vi "Boiler.vi"() -> ()   [LabVIEW 2016]
uses:
  Controls/Boiler Controls.ctl
  Controls/Boiler Simulation Controls.ctl
  Controls/Boiler Status Indicators.ctl
  Controls/States.ctl
  <vilib>/Utility/file.llb/Write Delimited Spreadsheet (string).vi
panel:
  in  "Stop the Application":bool
  out "Boiler Status Indicators":T1 {"Time Count" format="%.2g"}
  in  "Boiler Simulation Controls":T2 {"Flame Sensor Value (%)" min=0.0 max=100.0 scale=0.0..100.0}
  in  "Boiler Controls":T3 {"Fuel Valve Position" min=0.0 max=100.0 scale=0.0..100.0 scale format="%.2f"}
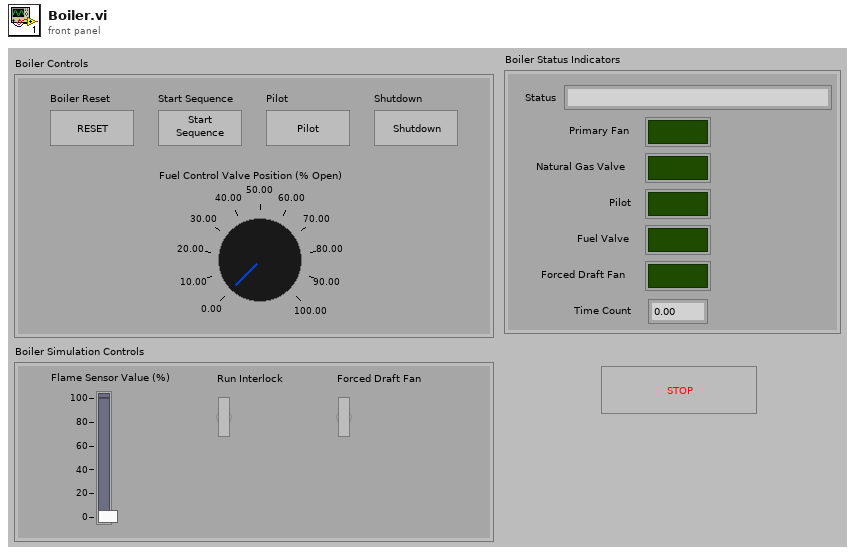
[diagram p1: front panel]
types:
  T1 = typedef "Boiler Status Indicators.ctl" = cluster{"Status":string, "Primary Fan":bool, "Natural Gas Valve":bool, "Pilot":bool, "Fuel Valve":bool, "Forced Draft Fan":bool, "Time Count":dbl}
  T2 = typedef "Boiler Simulation Controls.ctl" = cluster{"Flame Sensor Value (%)":dbl, "Run Interlock":bool, "Forced Draft Fan":bool}
  T3 = typedef "Boiler Controls.ctl" = cluster{"Boiler Reset":bool, "Start Sequence":bool, "Pilot":bool, "Shutdown":bool, "Fuel Valve Position":dbl}
  T4 = cluster{"Event string":string, "Event data string":string}
  T5 = typedef "States.ctl" = enum16{"Init", "Run", "Prove the Pilot", "Start and Run", "Shutdown"}
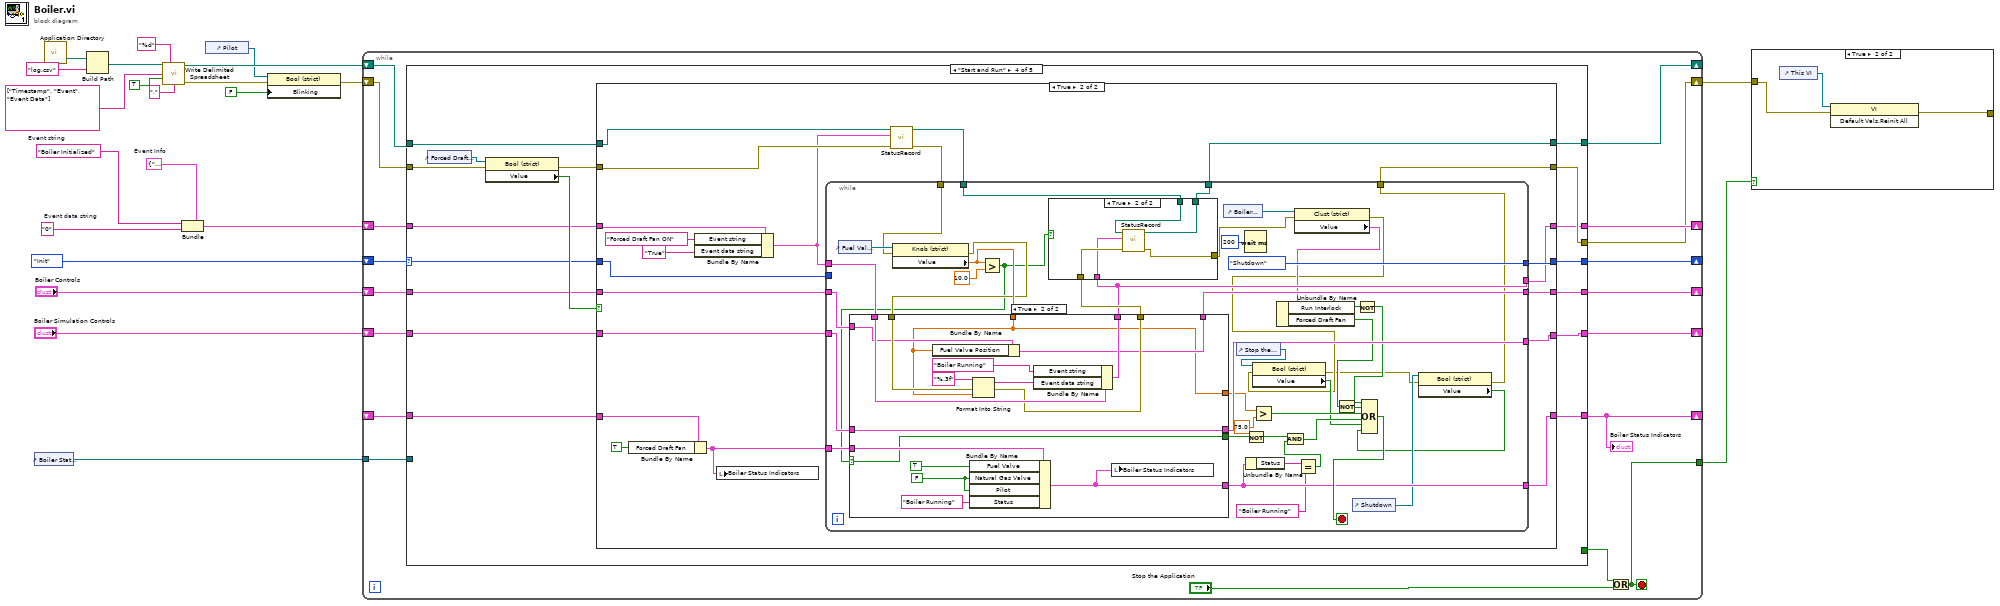
[diagram p0: block diagram]
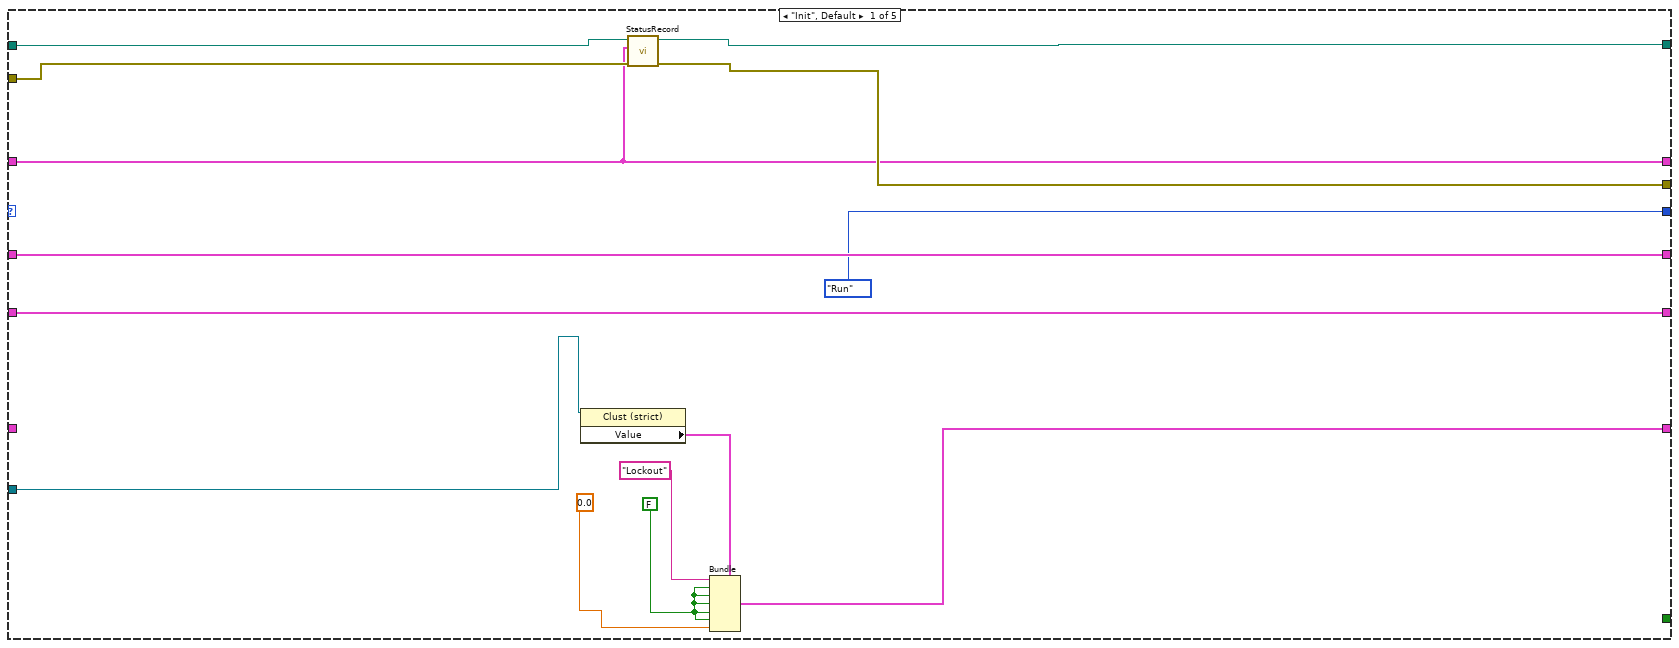
[diagram p3: hidden frame]
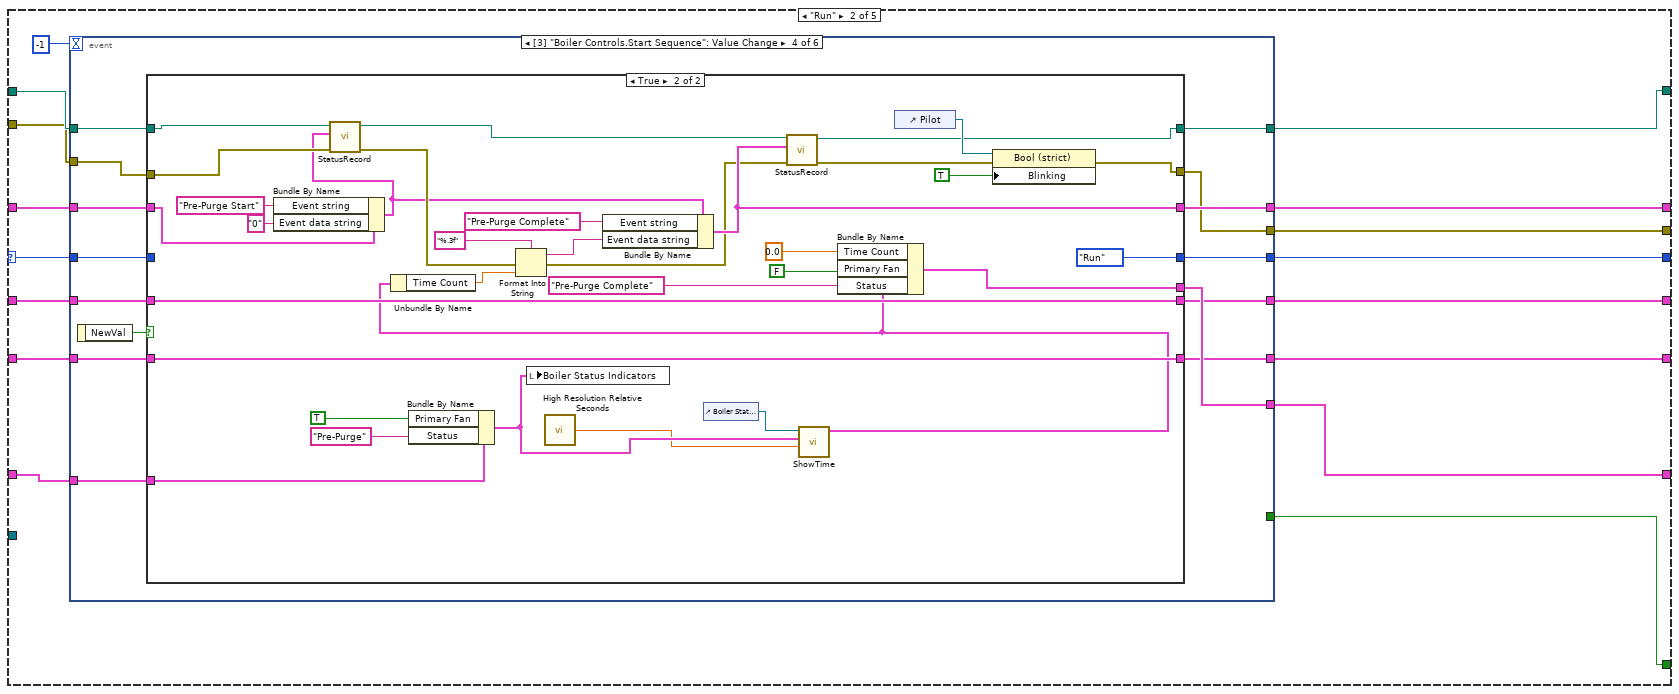
[diagram p4: hidden frame]
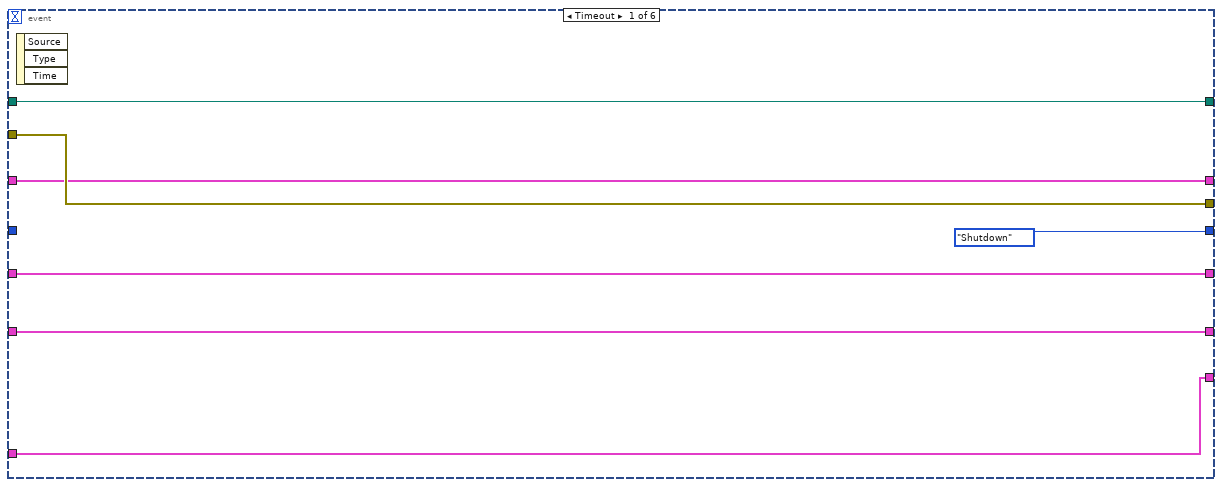
[diagram p5: hidden frame]
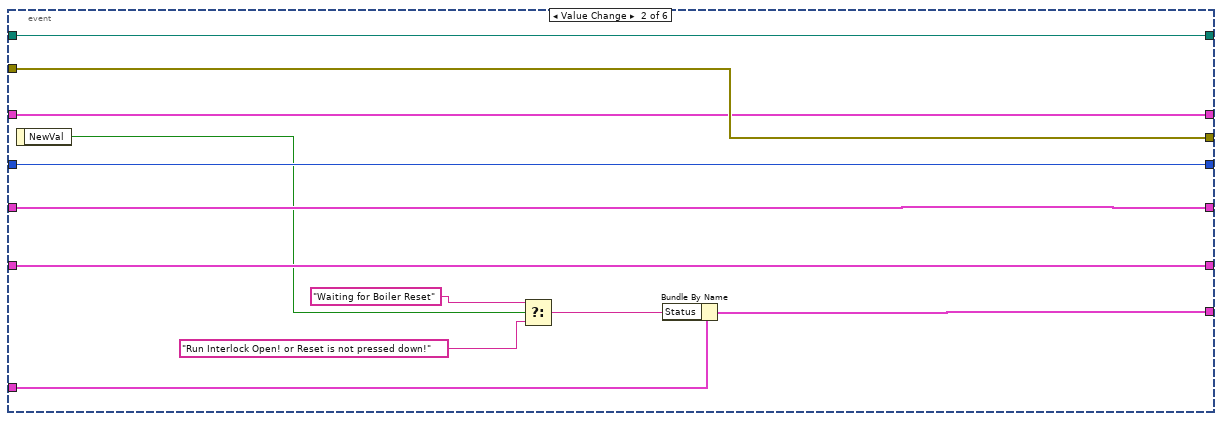
[diagram p6: hidden frame]
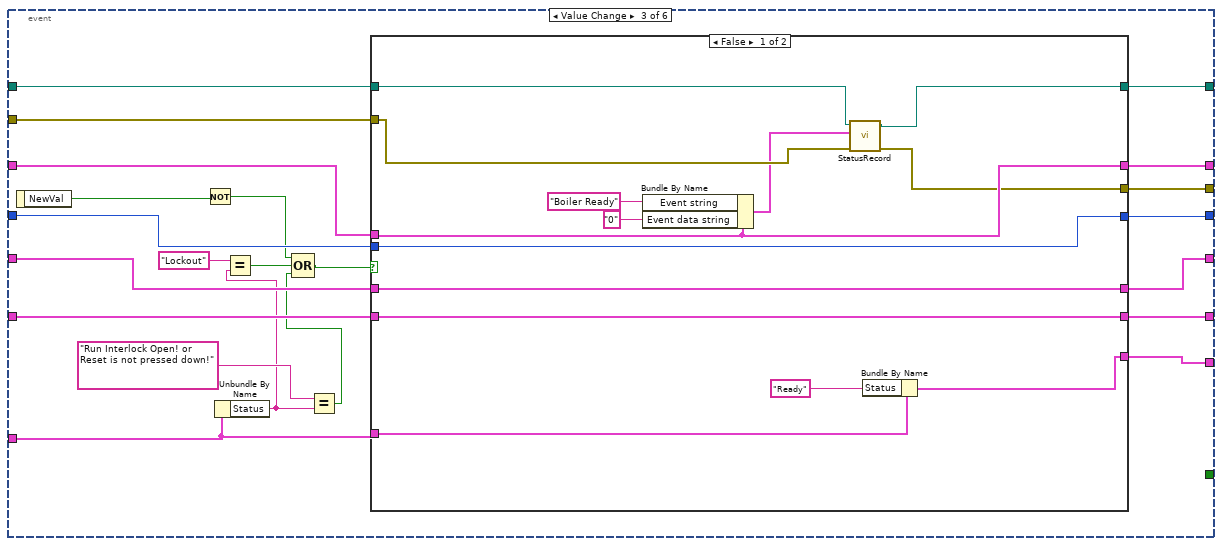
[diagram p7: hidden frame]
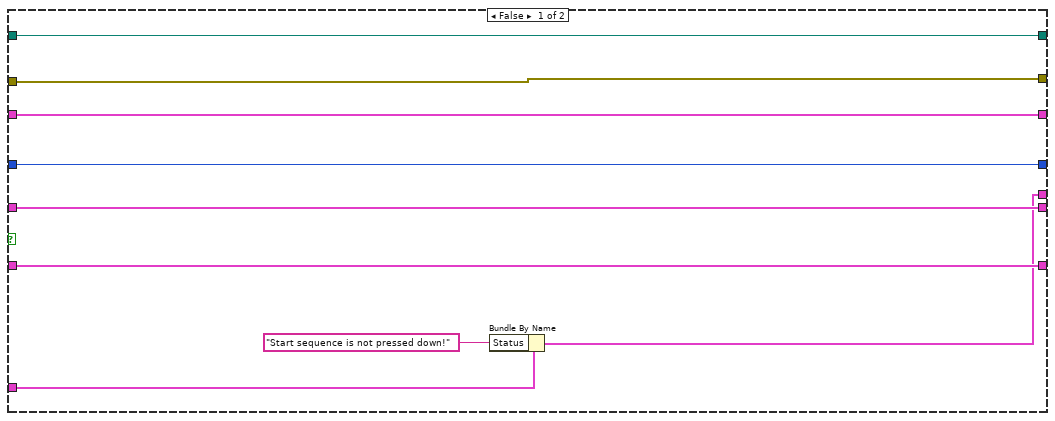
[diagram p9: hidden frame]
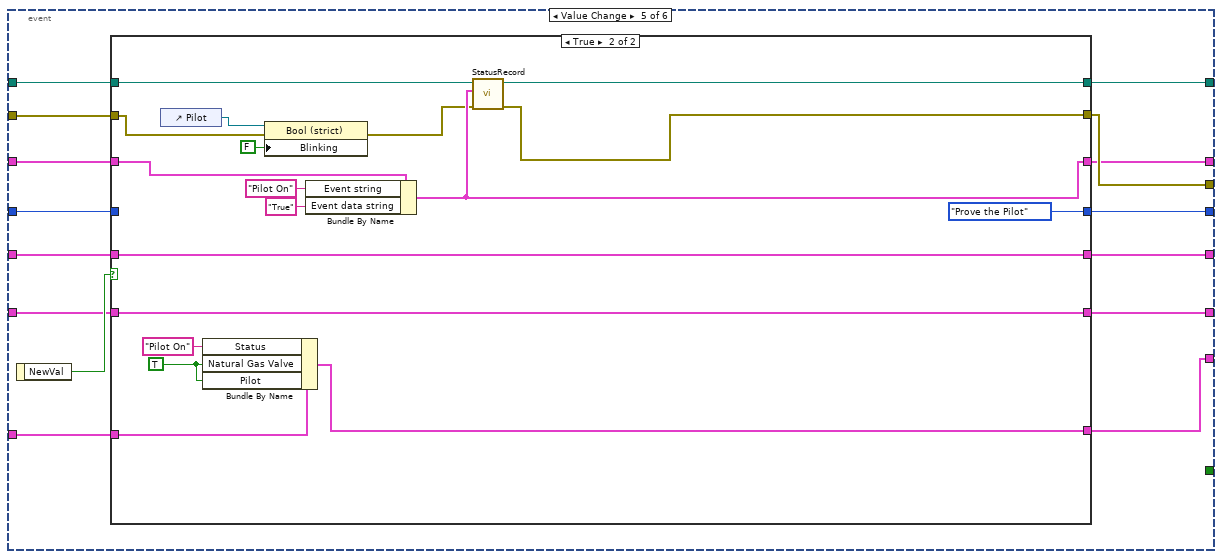
[diagram p10: hidden frame]
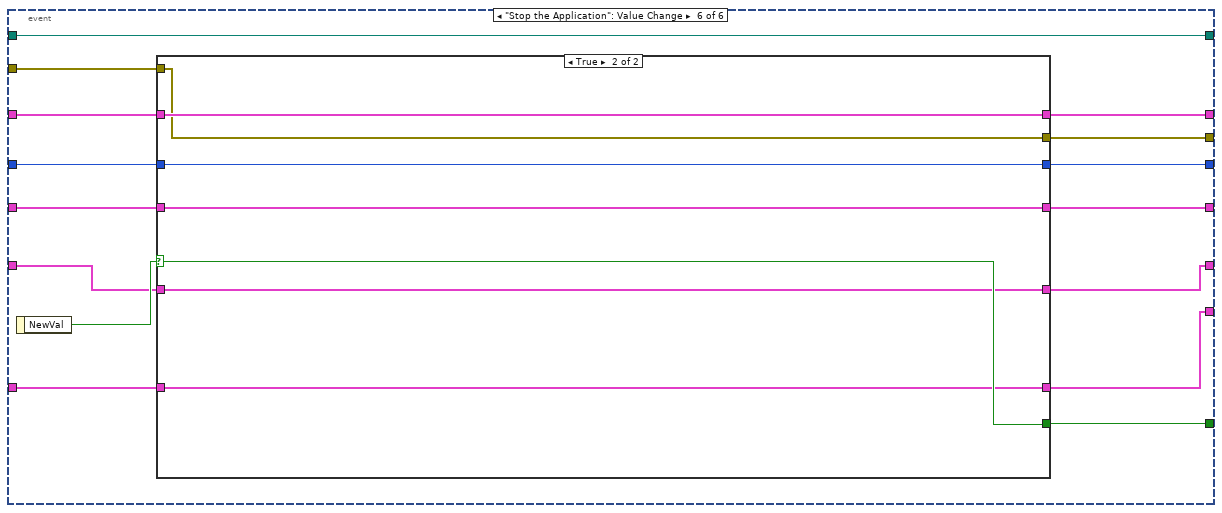
[diagram p12: hidden frame]
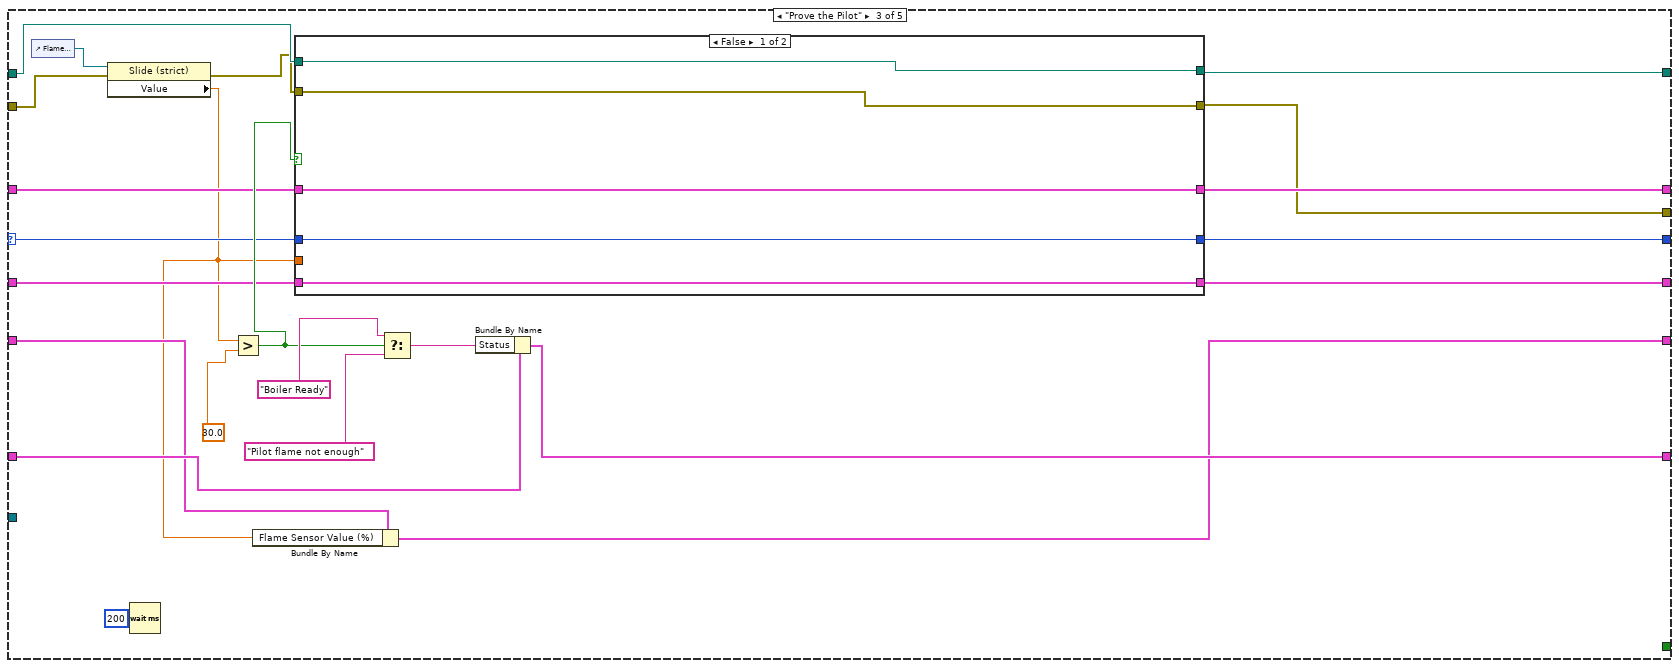
[diagram p14: hidden frame]
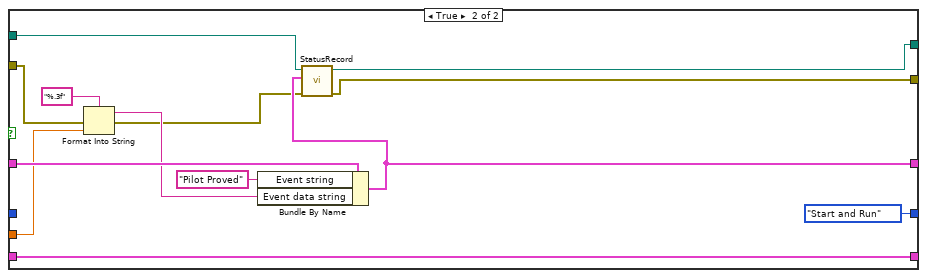
[diagram p15: hidden frame]
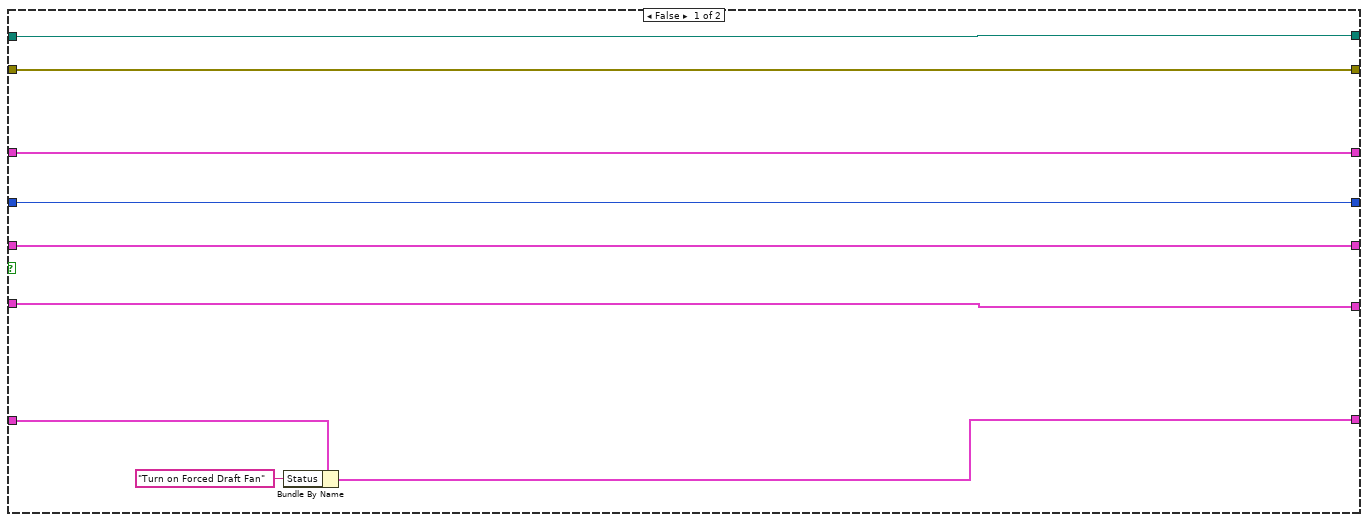
[diagram p16: hidden frame]
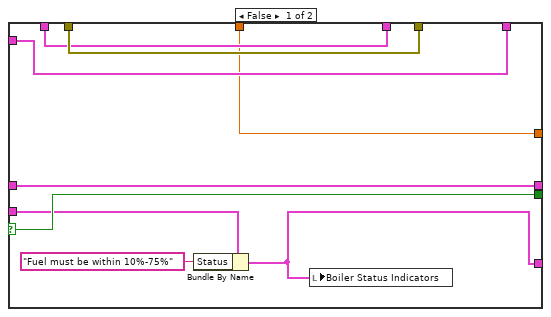
[diagram p18: hidden frame]
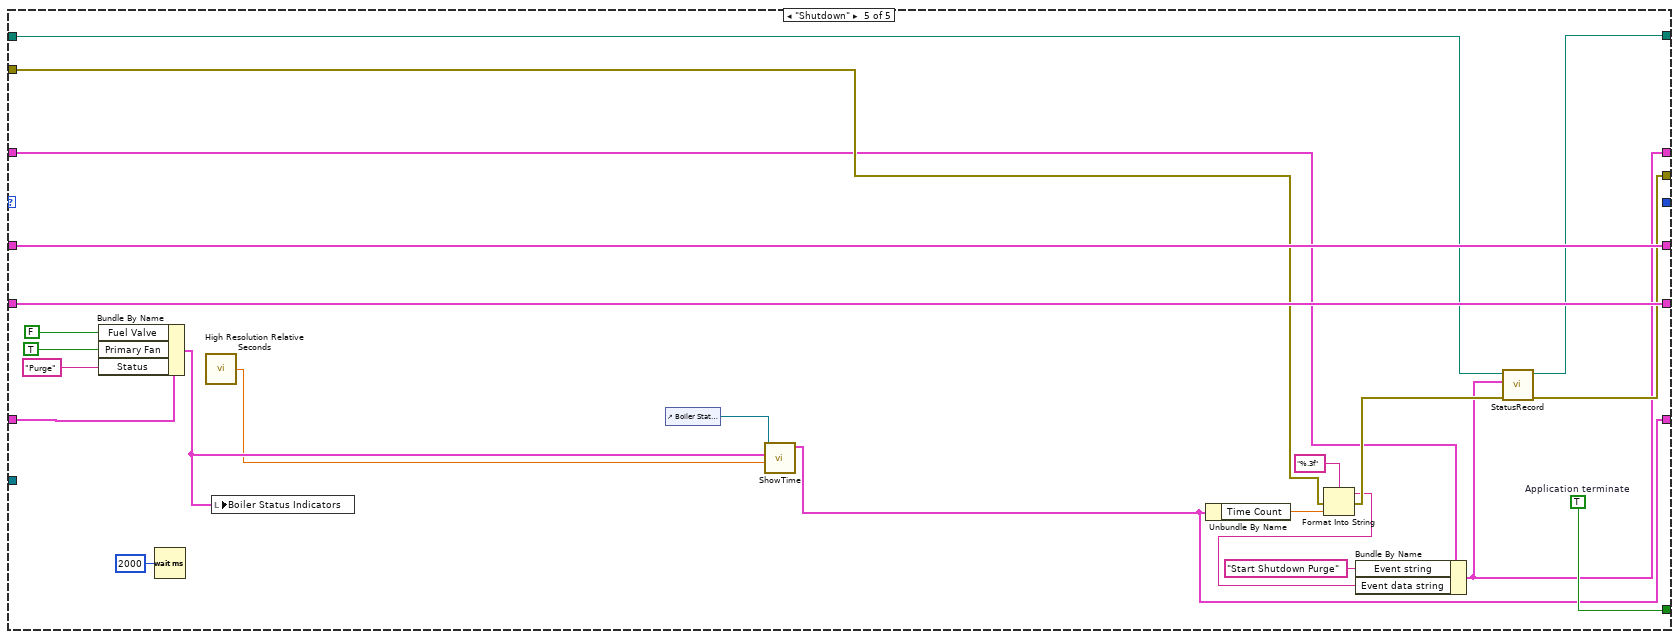
[diagram p19: hidden frame]
diagram:
  w7 = T4 {"Event string"="", "Event data string"=""}  # Event Info
  w17 = "Boiler Initialized"  # Event string
  w16 = "0"  # Event data string
  n1 = control-ref of="Boiler Status Indicators"() -> (w21:refnum<vi>)
  n2 = call <vilib>:"Application Directory.vi"() -> ("Application Directory"=w15:path)
  n3 = Build Path(base path=w15, name or relative path="log.csv") -> (appended path=w13:path)
  n4 = call-poly <vilib>:"Write Delimited Spreadsheet.vi"("file path (dialog if empty)"=w13, "format (%s)"="%d" ("format (%.3f)"), "1D data"=string[] ["Timestamp", "Event", "Event Data"], "append to file? (new file:F)"=TRUE, "delimiter (\\t)"="," ("delimiter (\\t)")) -> ("new file path (Not A Path if cancelled)"=w9:path, "error out"=w4:errorcluster)  [unwired: 9 in]
  n5 = Bundle(cluster=w7, "Event string"=w17, "Event data string"=w16) -> (w18:T4)
  n6 = control-ref of="Pilot"() -> (w5:refnum<vi>)
  n7 = property class="Bool (strict)"(reference=w5, error in=w4, "Blinking"=FALSE) -> (error out=w6:errorcluster)  [unwired: 1 out]
  n8 = while {
    tunnel: w21 -> [w39]
    shift-right: [w36] -> _
    shift-left: States."Init" -> [w40]
    shift-right: [w24] -> w2
    shift-left: w6 -> [w27]
    shift-right: [w34] -> _
    shift-left: w18 -> [w35]
    shift-right: [w31] -> _
    shift-left: "Boiler Controls" -> [w38]
    shift-right: [w32] -> _
    shift-left: "Boiler Simulation Controls" -> [w37]
    shift-right: [w25] -> _
    shift-left: _ -> [w30]
    shift-right: [w28] -> _
    shift-left: w9 -> [w29]
    tunnel: [w23] -> w1
    stop <- w23 stop-if-true
    n9 = case shown="\"Start and Run\"" w40 {
      selector: w40 -> [_ w64 w272 w307 _]
      tunnel: [w46 w59 w276 w300 w425] -> w25
      tunnel: w39 -> [w54 _ _ _ _]
      tunnel: w38 -> [w48 w65 w271 w305 w443]
      tunnel: w37 -> [w49 w66 w261 w303 w444]
      tunnel: [w49 w63 w259 w302 w444] -> w32
      tunnel: [w48 w62 w270 w304 w443] -> w31
      tunnel: [States."Run" w67 w269 w306 _] -> w36
      tunnel: [w44 w61 w266 w310 w427] -> w24
      tunnel: w27 -> [w45 w68 w264 w316 w432]
      tunnel: w35 -> [w41 w70 w273 w309 w430]
      tunnel: [w41 w60 w268 w308 w426] -> w34
      tunnel: [_ w57 _ _ w445] -> w33
      tunnel: w30 -> [_ w58 w278 w301 w439]
      tunnel: w29 -> [w43 w69 w274 w313 w429]
      tunnel: [w42 w55 w267 w312 w428] -> w28
      frame "Init", Default {
        w51 = FALSE ("Boiler Reset")
        n10 = property class="Clust (strict)"(reference=w54) -> ("Value"=w53:T1)  [unwired: 1 in, 2 out]
        n11 = call "StatusRecord.vi"("error in (no error)"=w45, "Event Info"=w41, "new file path (Not A Path if cancelled) in"=w43) -> ("error out"=w44:errorcluster, "new file path (Not A Path if cancelled) out"=w42:path)  [unwired: 7 in]
        n12 = Bundle(cluster=w53, "Status"="Lockout", "Primary Fan"=w51, "Natural Gas Valve"=w51, "Pilot"=w51, "Fuel Valve"=w51, "Forced Draft Fan"=w51, "Time Count"=0.0 ("Fuel Valve Position")) -> (w46:T1)
      }
      frame "Run" {
        n13 = event shown="[3] \"Boiler Controls.Start Sequence\": Value Change" {
          selector: _ -> [_ _ _ _ _ _]
          dyn-events: _ -> [_ _ _ _ _ _]
          timeout: -1 -> [_ _ _ _ _ _]
          tunnel: w70 -> [w74 w86 w102 w138 w199 w239]
          tunnel: w69 -> [w76 w88 w98 w135 w203 w242]
          tunnel: w68 -> [w75 w87 w100 w133 w201 w241]
          tunnel: [w76 w88 w97 w134 w202 w242] -> w55
          tunnel: [States."Shutdown" w85 w103 w139 w196 w236] -> w67
          tunnel: w66 -> [w72 w83 w108 w144 w193 w233]
          tunnel: w65 -> [w73 w84 w106 w142 w195 w235]
          tunnel: w58 -> [w71 w89 w110 w146 w191 w231]
          tunnel: [w71 w82 w109 w145 w190 w230] -> w59
          tunnel: w64 -> [_ w85 w104 w140 w197 w237]
          tunnel: [w72 w83 w107 w143 w192 w232] -> w63
          tunnel: [w73 w84 w105 w141 w194 w234] -> w62
          tunnel: [w75 w87 w99 w136 w200 w240] -> w61
          tunnel: [w74 w86 w101 w137 w198 w238] -> w60
          tunnel: [_ _ _ _ _ w243] -> w57
          event Timeout {
            n14 = event-data() -> ()  [unwired: 1 in, 3 out]
          }
          event Value Change {
            n15 = event-data() -> ("NewVal"=w81:bool)  [unwired: 1 in]
            n16 = Select(t="Waiting for Boiler Reset" ("Status"), s=w81, f="Run Interlock Open! or Reset is not pressed down!" ("Status")) -> (s? t:f=w78:string)
            n17 = Bundle By Name(cluster=w89, "Status"=w78) -> (w82:T1)
          }
          event Value Change {
            n18 = event-data() -> ("NewVal"=w96:bool)  [unwired: 1 in]
            n19 = Not(x=w96) -> (.not. x?=w95:bool)
            n20 = Unbundle By Name(w110) -> ("Status"=w93:string)
            n21 = Equal?(x="Lockout", y=w93) -> (x = y?=w91:bool)
            n22 = Equal?(x="Run Interlock Open! or Reset is not pressed down!" ("Status"), y=w93) -> (x = y?=w94:bool)
            n23 = Compound Arithmetic op=OR(w95, w91, w94) -> (w90:bool)
            n24 = case shown="False" w90 {
              tunnel: w110 -> [w122 w126]
              tunnel: [w118 w126] -> w109
              tunnel: w108 -> [w121 w127]
              tunnel: [w121 w127] -> w107
              tunnel: w106 -> [w120 w128]
              tunnel: [w120 w128] -> w105
              tunnel: w104 -> [w117 w129]
              tunnel: [w117 w129] -> w103
              tunnel: w102 -> [w119 w130]
              tunnel: [w119 w130] -> w101
              tunnel: w100 -> [w114 w131]
              tunnel: [w115 w131] -> w99
              tunnel: w98 -> [w113 w132]
              tunnel: [w116 w132] -> w97
              frame False {
                n25 = Bundle By Name(cluster=w119, "Event string"="Boiler Ready", "Event data string"="0") -> (w112:T4)
                n26 = call "StatusRecord.vi"("error in (no error)"=w114, "Event Info"=w112, "new file path (Not A Path if cancelled) in"=w113) -> ("error out"=w115:errorcluster, "new file path (Not A Path if cancelled) out"=w116:path)  [unwired: 7 in]
                n27 = Bundle By Name(cluster=w122, "Status"="Ready") -> (w118:T1)
              }
              frame True {
              }
            }
          }
          event Value Change {
            n28 = event-data() -> ("NewVal"=w147:bool)  [unwired: 1 in]
            n29 = case shown="True" w147 {
              tunnel: w146 -> [w155 w187]
              tunnel: [w148 w175] -> w145
              tunnel: w144 -> [w154 w186]
              tunnel: [w154 w186] -> w143
              tunnel: w142 -> [w153 w185]
              tunnel: [w153 w185] -> w141
              tunnel: w140 -> [w152 _]
              tunnel: [w152 States."Run"] -> w139
              tunnel: [w151 w163] -> w137
              tunnel: w138 -> [w151 w178]
              tunnel: [w150 w170] -> w136
              tunnel: w133 -> [w150 w158]
              tunnel: [w149 w165] -> w134
              tunnel: w135 -> [w149 w161]
              frame False {
                n30 = Bundle By Name(cluster=w155, "Status"="Start sequence is not pressed down!") -> (w148:T1)
              }
              frame True {
                n31 = Bundle By Name(cluster=w178, "Event string"="Pre-Purge Start", "Event data string"="0") -> (w157:T4)
                n32 = call "StatusRecord.vi"("error in (no error)"=w158, "Event Info"=w157, "new file path (Not A Path if cancelled) in"=w161) -> ("error out"=w159:errorcluster, "new file path (Not A Path if cancelled) out"=w160:path)  [unwired: 7 in]
                n33 = Bundle By Name(cluster=w187, "Primary Fan"=TRUE, "Status"="Pre-Purge") -> (w168:T1)
                n34 = local write "Boiler Status Indicators"(w168) -> ()
                n35 = call <vilib>:"High Resolution Relative Seconds.vi"() -> ("relative seconds"=w167:dbl)
                n36 = control-ref of="Boiler Status Indicators"() -> (w169:refnum<vi>)
                n37 = call "ShowTime.vi"("relative seconds"=w167, "Value in"=w168, "Cluster in"=w169) -> ("Value out"=w166:T1)  [unwired: 8 in]
                n38 = Unbundle By Name(w166) -> ("Time Count"=w182:dbl)
                n39 = Format Into String(format string="%.3f", error in=w159, w182) -> (resulting string=w180:string, error out=w162:errorcluster)  [unwired: 1 in]
                n40 = Bundle By Name(cluster=w157, "Event string"="Pre-Purge Complete", "Event data string"=w180) -> (w163:T4)
                n41 = call "StatusRecord.vi"("error in (no error)"=w162, "Event Info"=w163, "new file path (Not A Path if cancelled) in"=w160) -> ("error out"=w164:errorcluster, "new file path (Not A Path if cancelled) out"=w165:path)  [unwired: 7 in]
                n42 = Bundle By Name(cluster=w166, "Time Count"=0.0, "Primary Fan"=FALSE, "Status"="Pre-Purge Complete") -> (w175:T1)
                n43 = control-ref of="Pilot"() -> (w172:refnum<vi>)
                n44 = property class="Bool (strict)"(reference=w172, error in=w164, "Blinking"=TRUE) -> (error out=w170:errorcluster)  [unwired: 1 out]
              }
            }
          }
          event Value Change {
            n45 = event-data() -> ("NewVal"=w204:bool)  [unwired: 1 in]
            n46 = case shown="True" w204 {
              tunnel: [w211 w212] -> w202
              tunnel: w203 -> [w211 w216]
              tunnel: [w210 w213] -> w200
              tunnel: w201 -> [w210 w227]
              tunnel: [w209 w215] -> w198
              tunnel: w199 -> [w209 w220]
              tunnel: [w205 States."Prove the Pilot"] -> w196
              tunnel: w197 -> [w205 _]
              tunnel: [w208 w219] -> w194
              tunnel: w195 -> [w208 w219]
              tunnel: [w207 w218] -> w192
              tunnel: w193 -> [w207 w218]
              tunnel: [w206 w224] -> w190
              tunnel: w191 -> [w206 w226]
              frame False {
              }
              frame True {
                w225 = TRUE ("Natural Gas Valve")
                n47 = control-ref of="Pilot"() -> (w229:refnum<vi>)
                n48 = Bundle By Name(cluster=w226, "Status"="Pilot On", "Natural Gas Valve"=w225, "Pilot"=w225) -> (w224:T1)
                n49 = property class="Bool (strict)"(reference=w229, error in=w227, "Blinking"=FALSE) -> (error out=w214:errorcluster)  [unwired: 1 out]
                n50 = Bundle By Name(cluster=w220, "Event string"="Pilot On", "Event data string"="True") -> (w215:T4)
                n51 = call "StatusRecord.vi"("error in (no error)"=w214, "Event Info"=w215, "new file path (Not A Path if cancelled) in"=w216) -> ("error out"=w213:errorcluster, "new file path (Not A Path if cancelled) out"=w212:path)  [unwired: 7 in]
              }
            }
          }
          event "Stop the Application": Value Change {
            n52 = event-data() -> ("NewVal"=w244:bool)  [unwired: 1 in]
            n53 = case shown="True" w244 {
              selector: w244 -> [w251 w258]
              tunnel: [w251 w258] -> w243
              tunnel: w241 -> [w250 w256]
              tunnel: [w250 w256] -> w240
              tunnel: [w249 w257] -> w238
              tunnel: w239 -> [w249 w257]
              tunnel: [w248 w255] -> w236
              tunnel: w237 -> [w248 w255]
              tunnel: [w247 w254] -> w234
              tunnel: w235 -> [w247 w254]
              tunnel: w233 -> [w246 w253]
              tunnel: [w246 w253] -> w232
              tunnel: [w245 w252] -> w230
              tunnel: w231 -> [w245 w252]
              frame False {
              }
              frame True {
              }
            }
          }
        }
      }
      frame "Prove the Pilot" {
        n54 = control-ref of="Flame Sensor Value (%)"() -> (w262:refnum<vi>)
        n55 = property class="Slide (strict)"(reference=w262, error in=w264) -> (error out=w263:errorcluster, "Value"=w260:dbl)  [unwired: 1 out]
        n56 = Wait (ms)(milliseconds to wait=u32 200) -> ()  [unwired: 1 out]
        n57 = Greater?(x=w260, y=30.0) -> (0:w275:bool)
        n58 = Bundle By Name(cluster=w261, "Flame Sensor Value (%)"=w260) -> (w259:T2)
        n59 = case shown="False" w275 {
          tunnel: w274 -> [w286 w287]
          tunnel: w263 -> [w285 w295]
          tunnel: w273 -> [w284 w299]
          tunnel: w272 -> [w283 _]
          tunnel: w271 -> [w282 w293]
          tunnel: w260 -> [_ w296]
          tunnel: [w282 w293] -> w270
          tunnel: [w283 States."Start and Run"] -> w269
          tunnel: [w284 w291] -> w268
          tunnel: [w286 w288] -> w267
          tunnel: [w285 w289] -> w266
          frame False {
          }
          frame True {
            n60 = Format Into String(format string="%.3f", error in=w295, w296) -> (resulting string=w294:string, error out=w290:errorcluster)  [unwired: 1 in]
            n61 = Bundle By Name(cluster=w299, "Event string"="Pilot Proved", "Event data string"=w294) -> (w291:T4)
            n62 = call "StatusRecord.vi"("error in (no error)"=w290, "Event Info"=w291, "new file path (Not A Path if cancelled) in"=w287) -> ("error out"=w289:errorcluster, "new file path (Not A Path if cancelled) out"=w288:path)  [unwired: 7 in]
          }
        }
        n63 = Select(t="Boiler Ready", s=w275, f="Pilot flame not enough") -> (s? t:f=w277:string)
        n64 = Bundle By Name(cluster=w278, "Status"=w277) -> (w276:T1)
      }
      frame "Start and Run" {
        n65 = control-ref of="Forced Draft Fan"() -> (w315:refnum<vi>)
        n66 = property class="Bool (strict)"(reference=w315, error in=w316) -> (error out=w311:errorcluster, "Value"=w314:bool)  [unwired: 1 out]
        n67 = case shown="True" w314 {
          tunnel: [w325 w337] -> w312
          tunnel: w313 -> [w325 w330]
          tunnel: w311 -> [w324 w329]
          tunnel: [w324 w336] -> w310
          tunnel: [w323 w333] -> w308
          tunnel: w309 -> [w323 w344]
          tunnel: w307 -> [w322 w341]
          tunnel: [w322 w335] -> w306
          tunnel: [w321 w334] -> w304
          tunnel: w305 -> [w321 w342]
          tunnel: [w320 w331] -> w302
          tunnel: w303 -> [w320 w343]
          tunnel: [w318 w332] -> w300
          tunnel: w301 -> [w319 w340]
          frame False {
            n68 = Bundle By Name(cluster=w319, "Status"="Turn on Forced Draft Fan") -> (w318:T1)
          }
          frame True {
            n69 = Bundle By Name(cluster=w340, "Forced Draft Fan"=TRUE) -> (w338:T1)
            n70 = Bundle By Name(cluster=w344, "Event string"="Forced Draft Fan ON", "Event data string"="True") -> (w328:T4)
            n71 = local write "Boiler Status Indicators"(w338) -> ()
            n72 = call "StatusRecord.vi"("error in (no error)"=w329, "Event Info"=w328, "new file path (Not A Path if cancelled) in"=w330) -> ("error out"=w326:errorcluster, "new file path (Not A Path if cancelled) out"=w327:path)  [unwired: 7 in]
            n73 = while {
              tunnel: w327 -> [w384]
              tunnel: w326 -> [w388]
              tunnel: w343 -> [w382]
              tunnel: w342 -> [w376]
              tunnel: w341 -> [_]
              tunnel: w338 -> [w385]
              tunnel: [w368] -> w332
              tunnel: [w348] -> w337
              tunnel: [w350] -> w336
              tunnel: w328 -> [w378]
              tunnel: [States."Shutdown"] -> w335
              tunnel: [w381] -> w331
              tunnel: [w375] -> w334
              tunnel: [w374] -> w333
              stop <- w369 stop-if-true
              n74 = control-ref of="Fuel Valve Position"() -> (w389:refnum<vi>)
              n75 = property class="Knob (strict)"(reference=w389, error in=w388) -> (error out=w379:errorcluster, "Value"=w380:dbl)  [unwired: 1 out]
              n76 = Greater?(x=w380, y=10.0) -> (0:w347:bool)
              n77 = case shown="True" w347 {
                selector: w347 -> [w405 w417]
                tunnel: w385 -> [w399 w422]
                tunnel: [w397 w418] -> w368
                tunnel: [w405 w417] -> w363
                tunnel: w382 -> [w404 w416]
                tunnel: [w404 w416] -> w381
                tunnel: w380 -> [w400 w406]
                tunnel: w379 -> [w403 w412]
                tunnel: w378 -> [w402 w411]
                tunnel: [w402 w410] -> w374
                tunnel: [w403 w409] -> w377
                tunnel: w376 -> [w401 w408]
                tunnel: [w401 w407] -> w375
                tunnel: [w400 w406] -> w356
                frame False {
                  n78 = Bundle By Name(cluster=w399, "Status"="Fuel must be within 10%-75%") -> (w397:T1)
                  n79 = local write "Boiler Status Indicators"(w397) -> ()
                }
                frame True {
                  w420 = FALSE ("Natural Gas Valve")
                  n80 = Bundle By Name(cluster=w408, "Fuel Valve Position"=w406) -> (w407:T3)
                  n81 = Bundle By Name(cluster=w422, "Fuel Valve"=TRUE, "Natural Gas Valve"=w420, "Pilot"=w420, "Status"="Boiler Running") -> (w418:T1)
                  n82 = Format Into String(format string="%.3f", error in=w412, w406) -> (resulting string=w415:string, error out=w409:errorcluster)  [unwired: 1 in]
                  n83 = Bundle By Name(cluster=w411, "Event string"="Boiler Running", "Event data string"=w415) -> (w410:T4)
                  n84 = local write "Boiler Status Indicators"(w418) -> ()
                }
              }
              n85 = case shown="True" w347 {
                tunnel: [w391 w393] -> w348
                tunnel: w384 -> [w391 w394]
                tunnel: w377 -> [w390 w396]
                tunnel: w374 -> [_ w395]
                tunnel: [w390 w392] -> w373
                frame False {
                }
                frame True {
                  n86 = call "StatusRecord.vi"("error in (no error)"=w396, "Event Info"=w395, "new file path (Not A Path if cancelled) in"=w394) -> ("error out"=w392:errorcluster, "new file path (Not A Path if cancelled) out"=w393:path)  [unwired: 7 in]
                }
              }
              n87 = control-ref of="Boiler Simulation Controls"() -> (w372:refnum<vi>)
              n88 = control-ref of="Stop the Application"() -> (w355:refnum<vi>)
              n89 = Wait (ms)(milliseconds to wait=u32 200) -> ()  [unwired: 1 out]
              n90 = Not(x=w363) -> (.not. x?=w362:bool)
              n91 = Unbundle By Name(w368) -> ("Status"=w367:string)
              n92 = Greater?(x=w356, y=75.0) -> (0:w370:bool)
              n93 = property class="Clust (strict)"(reference=w372, error in=w373) -> (error out=w353:errorcluster, "Value"=w371:T2)  [unwired: 1 out]
              n94 = property class="Bool (strict)"(reference=w355, error in=w353) -> (error out=w351:errorcluster, "Value"=w354:bool)  [unwired: 1 out]
              n95 = Unbundle By Name(w371) -> ("Run Interlock"=w360:bool, "Forced Draft Fan"=w357:bool)
              n96 = Equal?(x=w367, y="Boiler Running") -> (x = y?=w365:bool)
              n97 = And(x=w362, y=w365) -> (x .and. y?=w361:bool)
              n98 = Not(x=w357) -> (.not. x?=w358:bool)
              n99 = control-ref of="Shutdown"() -> (w352:refnum<vi>)
              n100 = Not(x=w360) -> (.not. x?=w359:bool)
              n101 = property class="Bool (strict)"(reference=w352, error in=w351) -> (error out=w350:errorcluster, "Value"=w349:bool)  [unwired: 1 out]
              n102 = Compound Arithmetic op=OR(w359, w358, w370, w361, w354, w349) -> (w369:bool)
            }
          }
        }
      }
      frame "Shutdown" {
        w445 = TRUE  # Application terminate
        n103 = Bundle By Name(cluster=w439, "Fuel Valve"=FALSE, "Primary Fan"=TRUE, "Status"="Purge") -> (w437:T1)
        n104 = Wait (ms)(milliseconds to wait=u32 2000) -> ()  [unwired: 1 out]
        n105 = call <vilib>:"High Resolution Relative Seconds.vi"() -> ("relative seconds"=w436:dbl)
        n106 = local write "Boiler Status Indicators"(w437) -> ()
        n107 = control-ref of="Boiler Status Indicators"() -> (w423:refnum<vi>)
        n108 = call "ShowTime.vi"("relative seconds"=w436, "Value in"=w437, "Cluster in"=w423) -> ("Value out"=w425:T1)  [unwired: 8 in]
        n109 = Unbundle By Name(w425) -> ("Time Count"=w434:dbl)
        n110 = Format Into String(format string="%.3f", error in=w432, w434) -> (resulting string=w424:string, error out=w431:errorcluster)  [unwired: 1 in]
        n111 = Bundle By Name(cluster=w430, "Event string"="Start Shutdown Purge", "Event data string"=w424) -> (w426:T4)
        n112 = call "StatusRecord.vi"("error in (no error)"=w431, "Event Info"=w426, "new file path (Not A Path if cancelled) in"=w429) -> ("error out"=w427:errorcluster, "new file path (Not A Path if cancelled) out"=w428:path)  [unwired: 7 in]
      }
    }
    "Boiler Status Indicators" <- w25
    n113 = Or(x=w33, y="Stop the Application") -> (x .or. y?=w23:bool)
  }
  n114 = case shown="True" w1 {
    tunnel: w2 -> [w446 w448]
    tunnel: [w446 w447] -> _
    frame False {
    }
    frame True {
      n115 = control-ref of="This VI"() -> (w449:refnum<vi>)
      n116 = invoke class="VI" method="Default Vals.Reinit All"(reference=w449, error in=w448) -> (error out=w447:errorcluster)  [unwired: 1 in, 2 out]
    }
  }
